vi "PPMS_Data_Recorder2.vi"(1 "Output Amp #1":dbl=1.0, 2 "Output Amp #2":dbl=1.0, 3 "Output Amp #3":dbl=1.0) -> (7 "X-Value":dbl, 8 "X-Value 2":dbl, 9 "Theta-Value":dbl, 10 "Theta-Value 2":dbl)   [LabVIEW 2021]
uses:
  <instrlib>/Stanford Research 830/Public/Data/Read (All Parameters).vi
  \\ad.monash.edu\home/User060/c-nhppms/Desktop/Matt Gebert/LabViewPrograms/3rd Party Drivers/QDI-PPMS/QDInstrument.dll
  3rd Party Drivers/QDI-PPMS/QDInstrument.dll
  <instrlib>/Stanford Research 830/Stanford Research 830.lvlib
panel:
  in  "Data Format String":string="%.12f"
  out "Actual Save Path":path
  in  "File Notes:":string
  in  "<File Name>.dat  (Don't add extension)":string
  in  "Data Save Path:":path=path "C:/Users/labpc/Documents/ProbeStation Users Data"
  in  "Record data to file?":bool
  out "Temperature":dbl
  out "Field":dbl
  out "PPMS Initialisation":bool
  in  "Remote":bool
  out "PPMS Chamber Status":i32(ring) items=["ChamberUnknown"=0, "PurgedAndSealed"=1, "VentedAndSealed"=2, "Sealed"=3, "Purging"=4, "Venting"=5, "PreHiVac"=6, "HighVac"=7, "PumpContinuous"=8, "VentContinuous"=9, "ChamberFailure"=15]
  in  "External Reference Trigger (0: Sine Zero Crossing)  2":u16(ring) items=["Sine Zero Crossing", "TTL Rising Edge", "TTL Falling Edge"]
  in  "External Reference Trigger (0: Sine Zero Crossing)":u16(ring) items=["Sine Zero Crossing", "TTL Rising Edge", "TTL Falling Edge"]
  in  "External Reference Trigger #2 (0: Sine Zero Crossing)":u16(ring) items=["Sine Zero Crossing", "TTL Rising Edge", "TTL Falling Edge"]
  out "SR830 #3 Sensitivity 3":dbl
  out "SR830 #3 Sensitivity 2":dbl
  out "SR830 #3 Sensitivity":dbl
  out "Sense\nOver 3":bool
  out "Sense\nUnder 3":bool
  out "Sense\nOver 2":bool
  out "Sense\nUnder 2":bool
  out "Sense Under":bool
  out "Sense Over":bool
  in  "Loop Timing (ms)":u32=500
  out "Reference Freq 3":dbl
  out "Theta-Value 3":dbl
  out "R-Value 3":dbl
  out "X-Value 3":dbl
  out "Reference Freq 2":dbl
  out "R-Value 2":dbl
  out "Reference Freq":dbl
  out "R-Value":dbl
  out "Device Intialization":T1
  in  "System #3 Enabled/Disabled":bool
  in  "SR830 #3":refnum<visa-resource-name>="GPIB0::10::INSTR"
  in  "SR830 #3 Input Connection":u16(ring) items=["Single-Ended Voltage", "Differential Voltage", "1 MOhm Current Gain", "100 MOhm Current Gain"]
  in  "SR830 #3\nInput Coupling":u16(ring) items=["AC", "DC"]
  in  "SR830 #3 Input \nShield Grounding":u16(ring) items=["Float", "Ground"]
  in  "SR830 #3 Input\nNotch Filter":u16(ring) items=["None", "Line Notch", "2x Line Notch", "Both Notch Filters"]
  in  "SR830 #3 Trigger Source":u16(ring) items=["Internal", "External"]
  in  "SR830 #3 Internal \nReference Frequency":dbl=17.0
  in  "SR830 #3 Detection Harm. Num.":dbl=1.0
  in  "SR830 #3 Reference Source":u16(ring) items=["External", "Internal"]
  in  "SR830 #3 Manual \nPhase":dbl
  in  "SR830 #3 \nAuto Phase":bool
  in  "SR830 #3 \nTime Constant":u16(ring)=9 items=["10 us", "30 us", "100 us", "300 us", "1 ms", "3 ms", "10 ms", "30 ms", "100 ms", "300 ms", "1 s", "3 s", "10 s", "30 s", "100 s", "300 s", "1 ks", "3 ks", "10 ks", "30 ks"]
  in  "SR830 #3 Low\nPass Filter Slope":u16(ring)=3 items=["6 dB/oct", "12 dB/oct", "18 db/oct", "24 dB/oct"]
  in  "SR830 #3\nSync Filter":bool
  in  "SR830 #3 \nDynamic Reserve":i16(ring)=1 items=["Auto Reserve"=-1, "High Reserve"=0, "Normal"=1, "Low Noise"=2]
  in  "SR830 #3 Initial\nSensitivity":i16(ring)=17 items=["Auto Gain"=-1, "2 nV/fA"=0, "5 nV/fA"=1, "10 nV/fA"=2, "20 nV/fA"=3, "50 nV/fA"=4, "100 nV/fA"=5, "200 nV/fA"=6, "500 nV/fA"=7, "1 uV/pA"=8, "2 uV/pA"=9, "5 uV/pA"=10, "10 uV/pA"=11, "20 uV/pA"=12, "50 uV/pA"=13, "100 uV/pA"=14, "200 uV/pA"=15, "500 uV/pA"=16, "1 mV/nA"=17, "2 mV/nA"=18, "5 mV/nA"=19, "10 mV/nA"=20, "20 mV/nA"=21, "50 mV/nA"=22, "100 mV/nA"=23, "200 mV/nA"=24, "500 mV/mA"=25, "1 V/uA"=26]
  in  "System #2 Enabled/Disabled":bool
  in  "SR830 #2":refnum<visa-resource-name>="GPIB0::10::INSTR"
  in  "SR830 #2 Input Connection":u16(ring)=1 items=["Single-Ended Voltage", "Differential Voltage", "1 MOhm Current Gain", "100 MOhm Current Gain"]
  in  "SR830 #2\nInput Coupling":u16(ring) items=["AC", "DC"]
  in  "SR830 #2 Input \nShield Grounding":u16(ring) items=["Float", "Ground"]
  in  "SR830 #2 Input\nNotch Filter":u16(ring) items=["None", "Line Notch", "2x Line Notch", "Both Notch Filters"]
  in  "SR830 #2 Trigger Source":u16(ring) items=["Internal", "External"]
  in  "SR830 #2 Internal \nReference Frequency":dbl=17.0
  in  "SR830 #2 Detection Harm. Num.":dbl=1.0
  in  "SR830 #2 Reference Source":u16(ring) items=["External", "Internal"]
  in  "SR830 #2 Manual \nPhase":dbl
  in  "SR830 #2 \nAuto Phase":bool
  in  "SR830 #2 \nTime Constant":u16(ring)=8 items=["10 us", "30 us", "100 us", "300 us", "1 ms", "3 ms", "10 ms", "30 ms", "100 ms", "300 ms", "1 s", "3 s", "10 s", "30 s", "100 s", "300 s", "1 ks", "3 ks", "10 ks", "30 ks"]
  in  "SR830 #2 Low\nPass Filter Slope":u16(ring)=3 items=["6 dB/oct", "12 dB/oct", "18 db/oct", "24 dB/oct"]
  in  "SR830 #2\nSync Filter":bool
  in  "SR830 #2 \nDynamic Reserve":i16(ring)=1 items=["Auto Reserve"=-1, "High Reserve"=0, "Normal"=1, "Low Noise"=2]
  in  "SR830 #2 Initial \nSensitivity":i16(ring)=17 items=["Auto Gain"=-1, "2 nV/fA"=0, "5 nV/fA"=1, "10 nV/fA"=2, "20 nV/fA"=3, "50 nV/fA"=4, "100 nV/fA"=5, "200 nV/fA"=6, "500 nV/fA"=7, "1 uV/pA"=8, "2 uV/pA"=9, "5 uV/pA"=10, "10 uV/pA"=11, "20 uV/pA"=12, "50 uV/pA"=13, "100 uV/pA"=14, "200 uV/pA"=15, "500 uV/pA"=16, "1 mV/nA"=17, "2 mV/nA"=18, "5 mV/nA"=19, "10 mV/nA"=20, "20 mV/nA"=21, "50 mV/nA"=22, "100 mV/nA"=23, "200 mV/nA"=24, "500 mV/mA"=25, "1 V/uA"=26]
  in  "SR830 #1 Initial\nSensitivity":i16(ring)=17 items=["Auto Gain"=-1, "2 nV/fA"=0, "5 nV/fA"=1, "10 nV/fA"=2, "20 nV/fA"=3, "50 nV/fA"=4, "100 nV/fA"=5, "200 nV/fA"=6, "500 nV/fA"=7, "1 uV/pA"=8, "2 uV/pA"=9, "5 uV/pA"=10, "10 uV/pA"=11, "20 uV/pA"=12, "50 uV/pA"=13, "100 uV/pA"=14, "200 uV/pA"=15, "500 uV/pA"=16, "1 mV/nA"=17, "2 mV/nA"=18, "5 mV/nA"=19, "10 mV/nA"=20, "20 mV/nA"=21, "50 mV/nA"=22, "100 mV/nA"=23, "200 mV/nA"=24, "500 mV/mA"=25, "1 V/uA"=26]
  in  "SR830 #1 \nDynamic Reserve":i16(ring)=1 items=["Auto Reserve"=-1, "High Reserve"=0, "Normal"=1, "Low Noise"=2]
  in  "SR830 #1\nSync Filter":bool
  in  "SR830 #1 Low\nPass Filter Slope":u16(ring)=3 items=["6 dB/oct", "12 dB/oct", "18 db/oct", "24 dB/oct"]
  in  "SR830 #1 \nTime Constant":u16(ring)=8 items=["10 us", "30 us", "100 us", "300 us", "1 ms", "3 ms", "10 ms", "30 ms", "100 ms", "300 ms", "1 s", "3 s", "10 s", "30 s", "100 s", "300 s", "1 ks", "3 ks", "10 ks", "30 ks"]
  in  "SR830 #1 \nAuto Phase":bool
  in  "SR830 #1 Manual \nPhase":dbl
  in  "SR830 #1 Reference Source":u16(ring)=1 items=["External", "Internal"]
  in  "SR830 #1 Detection Harm. Num.":dbl=1.0
  in  "SR830 #1 Internal \nReference Frequency":dbl=17.0
  in  "SR830 #1 Trigger Source":u16(ring) items=["Internal", "External"]
  in  "SR830 #1 Input\nNotch Filter":u16(ring) items=["None", "Line Notch", "2x Line Notch", "Both Notch Filters"]
  in  "SR830 #1 Input \nShield Grounding":u16(ring) items=["Float", "Ground"]
  in  "SR830 #1\nInput Coupling":u16(ring) items=["AC", "DC"]
  in  "SR830 #1 Input Connection":u16(ring)=1 items=["Single-Ended Voltage", "Differential Voltage", "1 MOhm Current Gain", "100 MOhm Current Gain"]
  in  "SR830 #1":refnum<visa-resource-name>="GPIB0::10::INSTR"
  in  "System #1 Enabled/Disabled":bool
  in  "System Reset All?":bool
  in  "program_stop":bool
  out "Y-Value 3":dbl
  out "Y-Value 2":dbl
  out "Y-Value":dbl
  # "Readout (Recorded)"
  # "SR830"
  # "SR830"
  # "SR830"
  # "Input Signal"
  # "Input Signal"
  # "Input Signal"
  # "Readout (Recorded)"
  # "Readout (Recorded)"
  # "Source / Reference"
  # "Source / Reference"
  # "Source / Reference"
  # "Input Filters & Sens"
  # "Input Filters & Sens"
  # "Input Filters & Sens"
  # "Initialisation:\n--> Reset \n--> Instruments?"
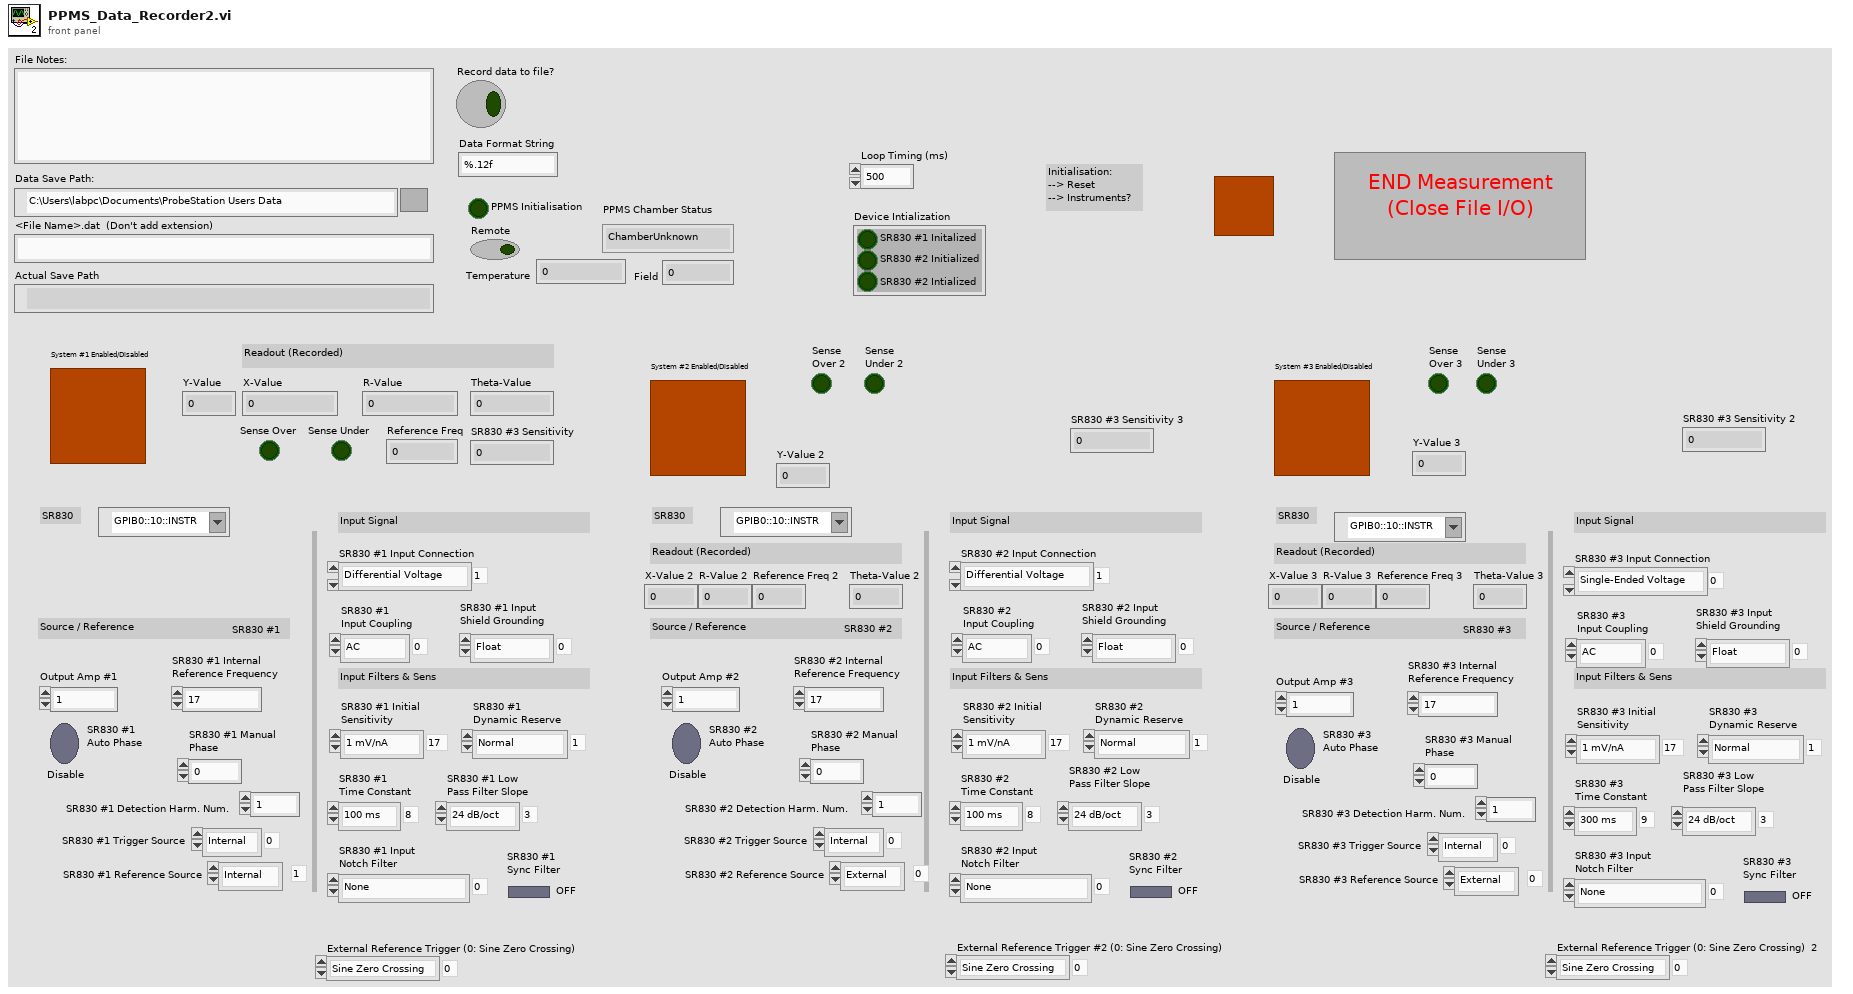
[diagram p1: front panel]
types:
  T1 = cluster{"SR830 #1 Initalized":bool, "SR830 #2 Initialized":bool, "SR830 #2 Intialized":bool}
  T2 = cluster{"Instrument Ref Out":refnum<k24>, "error out":errorcluster}
  T3 = cluster{"VISA resource name out":refnum<visa-resource-name>, "error out":errorcluster}
  T4 = cluster{"Initialised?":bool, "Initialised?":bool, "Initialised?":bool}
  T5 = cluster{"RecordingInProgress":bool, "refnum out":refnum<file>, "error out":errorcluster, "Actual Save Path":path}
  T6 = cluster{"Reference & Errors":cluster{"VISA resource name out":refnum<visa-resource-name>, "error out":errorcluster}, "Reference & Errors":cluster{"VISA resource name out":refnum<visa-resource-name>, "error out":errorcluster}, "Reference & Errors":cluster{"VISA resource name out":refnum<visa-resource-name>, "error out":errorcluster}}
  T7 = cluster{"Voltage Output":dbl, "Voltage Output":dbl, "Voltage Output":dbl}
  T8 = cluster{"Sensitivity":i16, "Sensitivity":i16, "Sensitivity":i16}
  T9 = cluster{"System #1 Enabled/Disabled":bool, "System #2 Enabled/Disabled":bool, "System #3 Enabled/Disabled":bool}
  T10 = cluster{"X-Value":dbl, "Y-Value":dbl, "R-Value":dbl, "Theta-Value":dbl, "Aux In 1 Value":dbl, "Aux In 2 Value":dbl, "Aux In 3 Value":dbl, "Aux In 4 Value":dbl, "Reference Frequency":dbl, "Channel 1 Display":dbl, "Channel 2 Display":dbl}
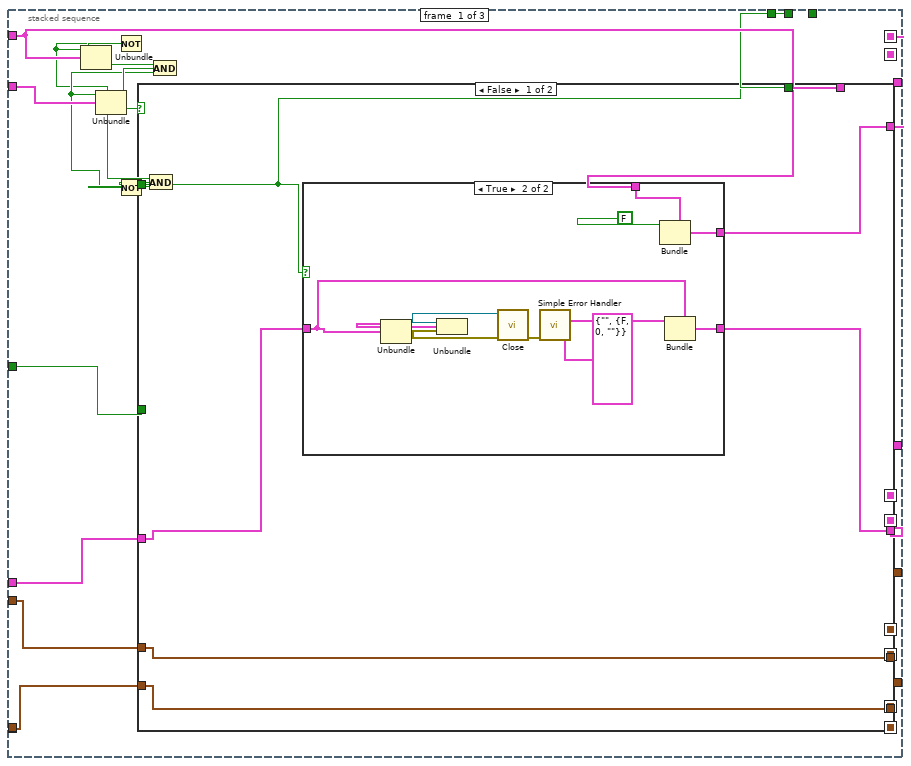
[diagram p6: hidden frame]
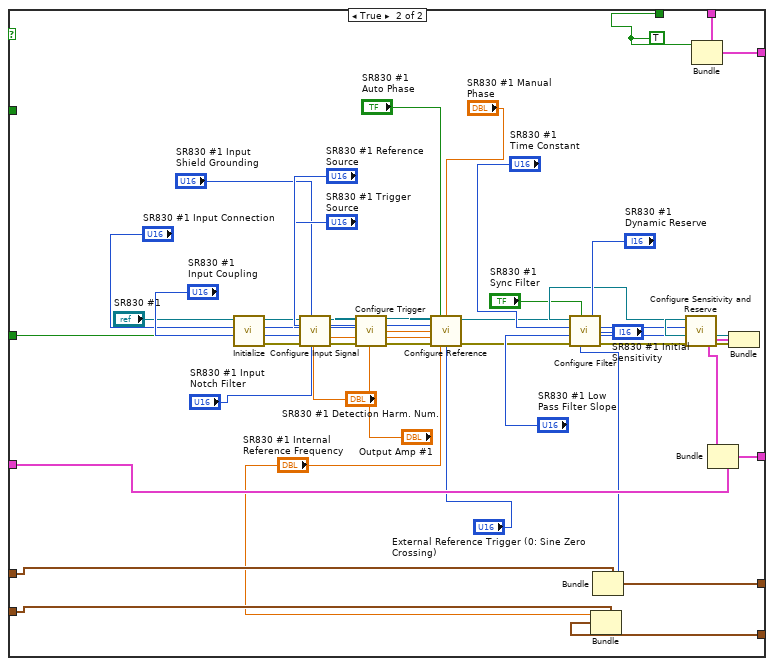
[diagram p8: hidden frame]
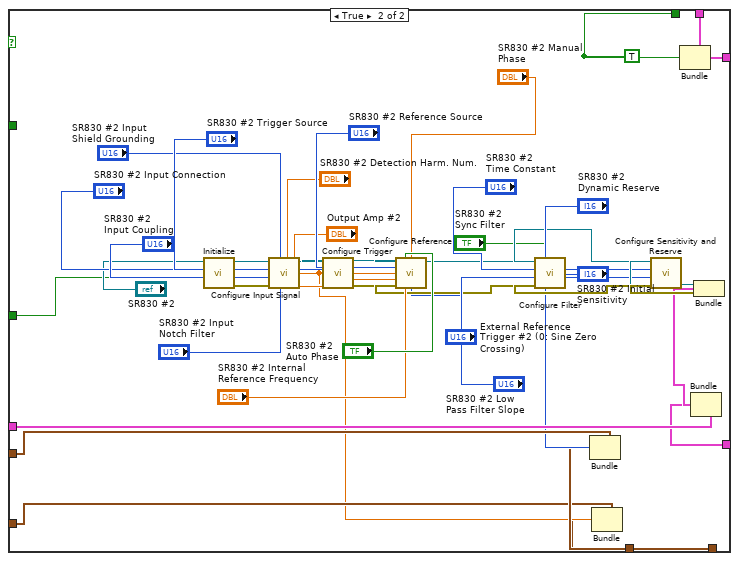
[diagram p10: hidden frame]
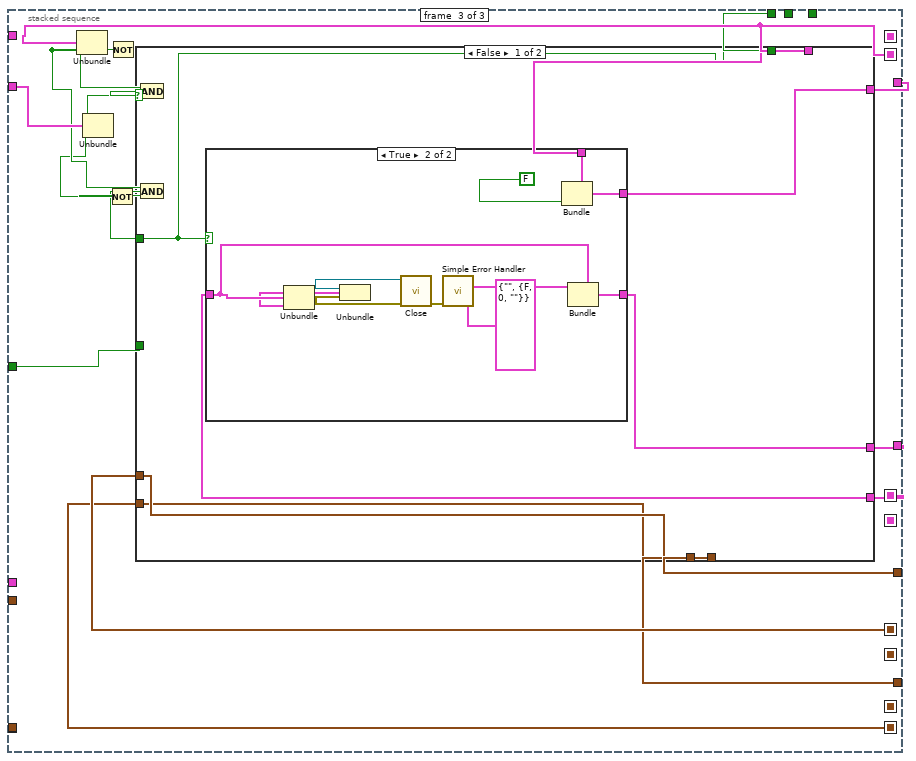
[diagram p11: hidden frame]
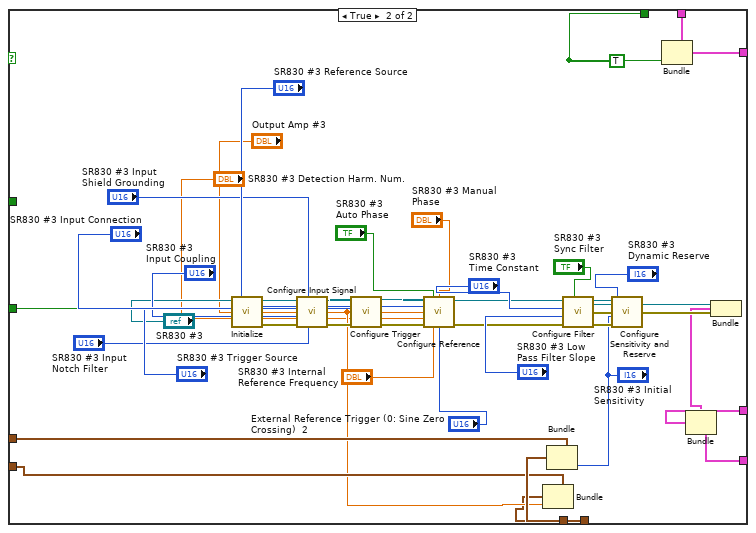
[diagram p13: hidden frame]
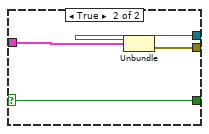
[diagram p14: hidden frame]
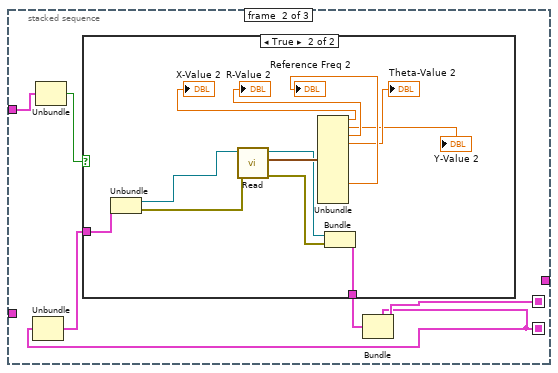
[diagram p16: hidden frame]
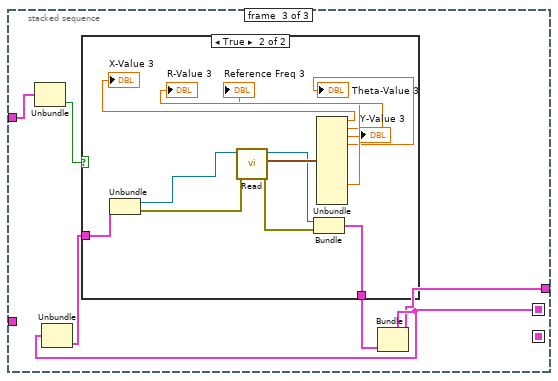
[diagram p18: hidden frame]
diagram:
  w5 = path ""  # Actual Save Path
  w9 = FALSE  # RecordingInProgress
  (unwired) FALSE  # File Init
  w10 = T2 {"Instrument Ref Out"=refnum, "error out"={"status"=FALSE, "code"=0, "source"=""}}  # PPMS Status Cluster
  w11 = FALSE  # PPMS Init
  w14 = 0.0 ("Voltage Output")
  w15 = i16 17 items=["Auto Gain"=-1, "2 nV/fA"=0, "5 nV/fA"=1, "10 nV/fA"=2, "20 nV/fA"=3, "50 nV/fA"=4, "100 nV/fA"=5, "200 nV/fA"=6, "500 nV/fA"=7, "1 uV/pA"=8, "2 uV/pA"=9, "5 uV/pA"=10, "10 uV/pA"=11, "20 uV/pA"=12, "50 uV/pA"=13, "100 uV/pA"=14, "200 uV/pA"=15, "500 uV/pA"=16, "1 mV/nA"=17, "2 mV/nA"=18, "5 mV/nA"=19, "10 mV/nA"=20, "20 mV/nA"=21, "50 mV/nA"=22, "100 mV/nA"=23, "200 mV/nA"=24, "500 mV/mA"=25, "1 V/uA"=26] ("Sensitivity")
  w25 = T3 {"VISA resource name out"="", "error out"={"status"=FALSE, "code"=0, "source"=""}} ("Reference & Errors")
  w27 = FALSE ("Initialised?")
  (unwired) ".txt"
  (unwired) FALSE ("Measuring")
  n1 = Bundle("Initialised?"=w27, "Initialised?"=w27, "Initialised?"=w27) -> (w26:T4)  [unwired: 1 in]
  n2 = Bundle("RecordingInProgress"=w9, "refnum out"=refnum<file> refnum, "error out"=errorcluster {"status"=FALSE, "code"=0, "source"=""}, "Actual Save Path"=w5) -> (w8:T5)  [unwired: 1 in]
  n3 = Bundle("Reference & Errors"=w25, "Reference & Errors"=w25, "Reference & Errors"=w25) -> (w24:T6)  [unwired: 1 in]
  n4 = Bundle("Voltage Output"=w14, "Voltage Output"=w14, "Voltage Output"=w14) -> (w13:T7)  [unwired: 1 in]
  n5 = Bundle("Sensitivity"=w15, "Sensitivity"=w15, "Sensitivity"=w15) -> (w12:T8)  [unwired: 1 in]
  n6 = while {
    shift-right: [w59] -> w23
    shift-left: w26 -> [w62]
    shift-right: [w48] -> w22
    shift-left: w24 -> [w47]
    shift-right: [w56] -> _
    shift-left: w12 -> [w58]
    shift-right: [w49] -> _
    shift-left: w13 -> [w53]
    shift-right: [w45] -> _
    shift-left: w11 -> [w46]
    shift-right: [w41] -> _
    shift-left: w10 -> [w43]
    shift-right: [w29] -> w4
    shift-left: w8 -> [w30]
    stop <- "program_stop" stop-if-true
    n7 = flat-sequence {
      tunnel: w62 -> [w80]
      tunnel: w47 -> [w79]
      tunnel: [w77] -> w61
      tunnel: [w78] -> w60
      tunnel: [w78] -> w59
      tunnel: w58 -> [w76]
      tunnel: [w75] -> w57
      tunnel: w53 -> [w74]
      tunnel: [w73] -> w52
      tunnel: w46 -> [w68]
      tunnel: [w67] -> w45
      tunnel: w43 -> [w66]
      tunnel: [w65] -> w42
      tunnel: [w64] -> w32
      tunnel: w61 -> [w374]
      tunnel: w60 -> [w373]
      tunnel: [w375] -> w40
      tunnel: w57 -> [w377]
      tunnel: [w377] -> w38
      tunnel: [w373] -> w36
      tunnel: w52 -> [w376]
      tunnel: [w376] -> w34
      tunnel: w42 -> [w372]
      tunnel: [w371] -> w41
      tunnel: w32 -> [w370]
      tunnel: [w370] -> w31
      tunnel: w40 -> [w457]
      tunnel: [w457] -> w39
      tunnel: w38 -> [w456]
      tunnel: [w456] -> w37
      tunnel: w36 -> [w450]
      tunnel: [w450] -> w35
      tunnel: w34 -> [w455]
      tunnel: [w455] -> w33
      tunnel: w31 -> [w454]
      tunnel: w30 -> [w449]
      tunnel: [w448] -> w29
      tunnel: w39 -> [w637]
      tunnel: w37 -> [w640]
      tunnel: [w640] -> w55
      tunnel: w35 -> [w638]
      tunnel: [w638] -> w54
      tunnel: w33 -> [w639]
      tunnel: [w636] -> w51
      tunnel: [w635] -> w50
      tunnel: w55 -> [w739]
      tunnel: [w738] -> w56
      tunnel: [w737] -> w48
      tunnel: w54 -> [w736]
      tunnel: w51 -> [w729]
      tunnel: w50 -> [w728]
      tunnel: [w728] -> w49
      frame #0 {
        # "Device Initialization or close"
        n8 = flat-sequence {
          tunnel: w80 -> [w97]
          tunnel: w79 -> [w96]
          tunnel: w76 -> [w93]
          tunnel: w74 -> [w91]
          tunnel: [w95] -> w72
          tunnel: [w94] -> w71
          tunnel: [w92] -> w70
          tunnel: [w90] -> w69
          tunnel: [w81] -> w64
          tunnel: [w339] -> w73
          tunnel: [w340] -> w75
          tunnel: [w341] -> w77
          tunnel: [w342] -> w78
          tunnel: w72 -> [w342]
          tunnel: w71 -> [w341]
          tunnel: w70 -> [w340]
          tunnel: w69 -> [w339]
          tunnel: w68 -> [w338]
          tunnel: [w337] -> w67
          tunnel: w66 -> [w331]
          tunnel: [w330] -> w65
          frame #0 {
            # "SR830 Lock In Amplifiers"
            n9 = Bundle("System #1 Enabled/Disabled"="System #1 Enabled/Disabled", "System #2 Enabled/Disabled"="System #2 Enabled/Disabled", "System #3 Enabled/Disabled"="System #3 Enabled/Disabled") -> (w87:T9)  [unwired: 1 in]
            n10 = stacked-sequence {
              seq-local: [w110 _ _] -> [_ w188 _]
              seq-local: [_ w187 _] -> [_ _ w265]
              seq-local: [w109 _ _] -> [_ w186 _]
              seq-local: [_ w185 _] -> [_ _ w263]
              seq-local: [w102 _ _] -> [_ w180 _]
              seq-local: [_ w179 _] -> [_ _ w257]
              seq-local: [_ w177 _] -> [_ _ w255]
              seq-local: [w100 _ _] -> [_ w178 _]
              tunnel: "System Reset All?" -> [w115 w192 w269]
              tunnel: w87 -> [w114 w191 w267]
              tunnel: w97 -> [w111 _ _]
              tunnel: w96 -> [w104 _ _]
              tunnel: [_ _ w264] -> w95
              tunnel: [_ _ w262] -> w94
              tunnel: w93 -> [w103 _ _]
              tunnel: [_ _ w256] -> w92
              tunnel: [w101 _ _] -> _
              tunnel: w91 -> [w101 _ _]
              tunnel: [_ _ w254] -> w90
              tunnel: [_ _ w253] -> w84
              tunnel: [w99 _ _] -> w83
              tunnel: [_ w176 _] -> w82
              frame #0 {
                n11 = Unbundle(w111) -> ("Initialised?"=w106:bool)  [unwired: 2 out]
                n12 = Unbundle(w114) -> ("System #1 Enabled/Disabled"=w107:bool)  [unwired: 2 out]
                n13 = Not(x=w106) -> (.not. x?=w113:bool)
                n14 = Not(x=w107) -> (.not. x?=w108:bool)
                n15 = And(x=w106, y=w108) -> (x .and. y?=w105:bool)
                n16 = And(x=w113, y=w107) -> (x .and. y?=w112:bool)
                n17 = case shown="False" w112 {
                  tunnel: w115 -> [_ w148]
                  tunnel: w111 -> [w120 w147]
                  tunnel: [w119 w146] -> w110
                  tunnel: w104 -> [w122 w145]
                  tunnel: [w121 w143] -> w109
                  tunnel: w105 -> [w116 _]
                  tunnel: w103 -> [w118 w142]
                  tunnel: [w118 w141] -> w102
                  tunnel: w101 -> [w117 w139]
                  tunnel: [w117 w138] -> w100
                  tunnel: [w116 w135] -> w99
                  frame False {
                    n18 = case shown="True" w116 {
                      tunnel: w122 -> [w124 w131]
                      tunnel: [w124 w129] -> w121
                      tunnel: w120 -> [w123 w126]
                      tunnel: [w123 w125] -> w119
                      frame False {
                      }
                      frame True {
                        n19 = Unbundle(w131) -> ("Reference & Errors"=w128:T3)  [unwired: 2 out]
                        n20 = Unbundle(w128) -> ("VISA resource name out"=w133:refnum<visa-resource-name>, "error out"=w132:errorcluster)
                        n21 = call <instrlib>:"Close.vi"("error in (no error)"=w132, "VISA resource name"=w133) -> ("error out"=w134:errorcluster)  [unwired: 9 in]
                        n22 = call <vilib>:"Simple Error Handler.vi"("error in (no error)"=w134) -> ()  [unwired: 4 in, 5 out]
                        n23 = Bundle(cluster=w126, "Initialised?"=FALSE) -> (w125:T4)  [unwired: 2 in]
                        n24 = Bundle(cluster=w131, "Reference & Errors"=T3 {"VISA resource name out"="", "error out"={"status"=FALSE, "code"=0, "source"=""}}) -> (w129:T6)  [unwired: 2 in]
                      }
                    }
                  }
                  frame True {
                    w135 = TRUE
                    n25 = call <instrlib>:"Initialize.vi"("Reset (True)"=w148, "VISA resource name"="SR830 #1") -> ("error out"=w153:errorcluster, "VISA resource name out"=w152:refnum<visa-resource-name>)  [unwired: 8 in]
                    n26 = call <instrlib>:"Configure Input Signal.vi"("Input Notch Filter (0: None)"="SR830 #1 Input\nNotch Filter", "Input Shield Grounding (0: Float)"="SR830 #1 Input \nShield Grounding", "error in (no error)"=w153, "Input Coupling (0: AC)"="SR830 #1\nInput Coupling", "Input Connection (0: Single-Ended Voltage)"="SR830 #1 Input Connection", "VISA resource name"=w152) -> ("error out"=w155:errorcluster, "VISA resource name out"=w154:refnum<visa-resource-name>)  [unwired: 4 in]
                    n27 = call <instrlib>:"Configure Trigger.vi"("error in (no error)"=w155, "Trigger Source (0: Internal)"="SR830 #1 Trigger Source", "VISA resource name"=w154) -> ("error out"=w157:errorcluster, "VISA resource name out"=w156:refnum<visa-resource-name>)  [unwired: 7 in]
                    n28 = call <instrlib>:"Configure Reference.vi"("VISA resource name"=w156, "Auto Phase (T: Enabled)"="SR830 #1 \nAuto Phase", "Manual Phase (0 Degree)"="SR830 #1 Manual \nPhase", "Reference Source (1: Internal)"="SR830 #1 Reference Source", "Sine Output Amplitude (1 V)"="Output Amp #1", "Detection Harmonic Number (1)"="SR830 #1 Detection Harm. Num.", "error in (no error)"=w157, "Internal Reference Frequency (1000 Hz)"="SR830 #1 Internal \nReference Frequency", "External Reference Trigger (0: Sine Zero Crossing)"="External Reference Trigger (0: Sine Zero Crossing)") -> ("VISA resource name out"=w159:refnum<visa-resource-name>, "error out"=w158:errorcluster)  [unwired: 5 in]
                    n29 = call <instrlib>:"Configure Filter.vi"("Enable Sync Filter (F: Disable)"="SR830 #1\nSync Filter", "error in (no error)"=w158, "Low Pass Filter Slope (1: 12dB/oct)"="SR830 #1 Low\nPass Filter Slope", "Time Constant (8: 100ms)"="SR830 #1 \nTime Constant", "VISA resource name"=w159) -> ("error out"=w172:errorcluster, "VISA resource name out"=w171:refnum<visa-resource-name>)  [unwired: 5 in]
                    n30 = Bundle(cluster=w139, "Voltage Output"="SR830 #1 Internal \nReference Frequency") -> (w138:T7)  [unwired: 2 in]
                    n31 = Bundle(cluster=w142, "Sensitivity"="SR830 #1 Initial\nSensitivity") -> (w141:T8)  [unwired: 2 in]
                    n32 = call <instrlib>:"Configure Sensitivity and Reserve.vi"("error in (no error)"=w172, "Sensitivity (-1: Auto gain)"="SR830 #1 Initial\nSensitivity", "Dynamic Reserve (-1: Auto Reserve)"="SR830 #1 \nDynamic Reserve", "VISA resource name"=w171) -> ("error out"=w175:errorcluster, "VISA resource name out"=w174:refnum<visa-resource-name>)  [unwired: 6 in]
                    n33 = Bundle(cluster=w147, "Initialised?"=w135) -> (w146:T4)  [unwired: 2 in]
                    n34 = Bundle("VISA resource name out"=w174, "error out"=w175) -> (w144:T3)  [unwired: 1 in]
                    n35 = Bundle(cluster=w145, "Reference & Errors"=w144) -> (w143:T6)  [unwired: 2 in]
                  }
                }
              }
              frame #1 {
                n36 = Unbundle(w188) -> ("Initialised?"=w182:bool)  [unwired: 2 out]
                n37 = Unbundle(w191) -> ("System #2 Enabled/Disabled"=w181:bool)  [unwired: 2 out]
                n38 = Not(x=w181) -> (.not. x?=w184:bool)
                n39 = And(x=w182, y=w184) -> (x .and. y?=w183:bool)
                n40 = Not(x=w182) -> (.not. x?=w190:bool)
                n41 = And(x=w190, y=w181) -> (x .and. y?=w189:bool)
                n42 = case shown="False" w189 {
                  tunnel: w192 -> [_ w225]
                  tunnel: w188 -> [w197 w224]
                  tunnel: [w196 w223] -> w187
                  tunnel: w186 -> [w199 w221]
                  tunnel: [w198 w220] -> w185
                  tunnel: w183 -> [w193 _]
                  tunnel: w180 -> [w195 w219]
                  tunnel: [w195 w217] -> w179
                  tunnel: w178 -> [w194 w216]
                  tunnel: [w194 w214] -> w177
                  tunnel: [w193 w212] -> w176
                  frame False {
                    n43 = case shown="True" w193 {
                      tunnel: w199 -> [w201 w208]
                      tunnel: [w201 w206] -> w198
                      tunnel: w197 -> [w200 w204]
                      tunnel: [w200 w203] -> w196
                      frame False {
                      }
                      frame True {
                        n44 = Unbundle(w208) -> ("Reference & Errors"=w205:T3)  [unwired: 2 out]
                        n45 = Unbundle(w205) -> ("VISA resource name out"=w210:refnum<visa-resource-name>, "error out"=w209:errorcluster)
                        n46 = call <instrlib>:"Close.vi"("error in (no error)"=w209, "VISA resource name"=w210) -> ("error out"=w211:errorcluster)  [unwired: 9 in]
                        n47 = call <vilib>:"Simple Error Handler.vi"("error in (no error)"=w211) -> ()  [unwired: 4 in, 5 out]
                        n48 = Bundle(cluster=w208, "Reference & Errors"=T3 {"VISA resource name out"="", "error out"={"status"=FALSE, "code"=0, "source"=""}}) -> (w206:T6)  [unwired: 2 in]
                        n49 = Bundle(cluster=w204, "Initialised?"=FALSE) -> (w203:T4)  [unwired: 2 in]
                      }
                    }
                  }
                  frame True {
                    w212 = TRUE
                    n50 = call <instrlib>:"Initialize.vi"("Reset (True)"=w225, "VISA resource name"="SR830 #2") -> ("error out"=w230:errorcluster, "VISA resource name out"=w229:refnum<visa-resource-name>)  [unwired: 8 in]
                    n51 = call <instrlib>:"Configure Input Signal.vi"("Input Notch Filter (0: None)"="SR830 #2 Input\nNotch Filter", "Input Shield Grounding (0: Float)"="SR830 #2 Input \nShield Grounding", "error in (no error)"=w230, "Input Coupling (0: AC)"="SR830 #2\nInput Coupling", "Input Connection (0: Single-Ended Voltage)"="SR830 #2 Input Connection", "VISA resource name"=w229) -> ("error out"=w232:errorcluster, "VISA resource name out"=w231:refnum<visa-resource-name>)  [unwired: 4 in]
                    n52 = call <instrlib>:"Configure Trigger.vi"("error in (no error)"=w232, "Trigger Source (0: Internal)"="SR830 #2 Trigger Source", "VISA resource name"=w231) -> ("error out"=w234:errorcluster, "VISA resource name out"=w233:refnum<visa-resource-name>)  [unwired: 7 in]
                    n53 = call <instrlib>:"Configure Reference.vi"("VISA resource name"=w233, "Auto Phase (T: Enabled)"="SR830 #2 \nAuto Phase", "Manual Phase (0 Degree)"="SR830 #2 Manual \nPhase", "Reference Source (1: Internal)"="SR830 #2 Reference Source", "Sine Output Amplitude (1 V)"="Output Amp #2", "Detection Harmonic Number (1)"="SR830 #2 Detection Harm. Num.", "error in (no error)"=w234, "Internal Reference Frequency (1000 Hz)"="SR830 #2 Internal \nReference Frequency", "External Reference Trigger (0: Sine Zero Crossing)"="External Reference Trigger #2 (0: Sine Zero Crossing)") -> ("VISA resource name out"=w236:refnum<visa-resource-name>, "error out"=w235:errorcluster)  [unwired: 5 in]
                    n54 = call <instrlib>:"Configure Filter.vi"("Enable Sync Filter (F: Disable)"="SR830 #2\nSync Filter", "error in (no error)"=w235, "Low Pass Filter Slope (1: 12dB/oct)"="SR830 #2 Low\nPass Filter Slope", "Time Constant (8: 100ms)"="SR830 #2 \nTime Constant", "VISA resource name"=w236) -> ("error out"=w249:errorcluster, "VISA resource name out"=w248:refnum<visa-resource-name>)  [unwired: 5 in]
                    n55 = Bundle(cluster=w219, "Sensitivity"="SR830 #2 Initial \nSensitivity") -> (w217:T8)  [unwired: 2 in]
                    n56 = Bundle(cluster=w216, "Voltage Output"="Output Amp #2") -> (w214:T7)  [unwired: 2 in]
                    n57 = call <instrlib>:"Configure Sensitivity and Reserve.vi"("error in (no error)"=w249, "Sensitivity (-1: Auto gain)"="SR830 #2 Initial \nSensitivity", "Dynamic Reserve (-1: Auto Reserve)"="SR830 #2 \nDynamic Reserve", "VISA resource name"=w248) -> ("error out"=w252:errorcluster, "VISA resource name out"=w251:refnum<visa-resource-name>)  [unwired: 6 in]
                    n58 = Bundle(cluster=w224, "Initialised?"=w212) -> (w223:T4)  [unwired: 2 in]
                    n59 = Bundle("VISA resource name out"=w251, "error out"=w252) -> (w222:T3)  [unwired: 1 in]
                    n60 = Bundle(cluster=w221, "Reference & Errors"=w222) -> (w220:T6)  [unwired: 2 in]
                  }
                }
              }
              frame #2 {
                n61 = Unbundle(w265) -> ("Initialised?"=w260:bool)  [unwired: 2 out]
                n62 = Unbundle(w267) -> ("System #3 Enabled/Disabled"=w259:bool)  [unwired: 2 out]
                n63 = Not(x=w259) -> (.not. x?=w261:bool)
                n64 = Not(x=w260) -> (.not. x?=w268:bool)
                n65 = And(x=w268, y=w259) -> (x .and. y?=w266:bool)
                n66 = And(x=w260, y=w261) -> (x .and. y?=w258:bool)
                n67 = case shown="False" w266 {
                  tunnel: w269 -> [_ w303]
                  tunnel: w265 -> [w274 w302]
                  tunnel: [w273 w301] -> w264
                  tunnel: w258 -> [w270 _]
                  tunnel: w263 -> [w276 w300]
                  tunnel: [w275 w299] -> w262
                  tunnel: w257 -> [w272 w297]
                  tunnel: [w272 w296] -> w256
                  tunnel: w255 -> [w271 w294]
                  tunnel: [w271 w292] -> w254
                  tunnel: [w270 w289] -> w253
                  frame False {
                    n68 = case shown="True" w270 {
                      tunnel: w276 -> [w278 w285]
                      tunnel: [w278 w283] -> w275
                      tunnel: w274 -> [w277 w281]
                      tunnel: [w277 w280] -> w273
                      frame False {
                      }
                      frame True {
                        n69 = Unbundle(w285) -> ("Reference & Errors"=w282:T3)  [unwired: 2 out]
                        n70 = Unbundle(w282) -> ("VISA resource name out"=w287:refnum<visa-resource-name>, "error out"=w286:errorcluster)
                        n71 = call <instrlib>:"Close.vi"("error in (no error)"=w286, "VISA resource name"=w287) -> ("error out"=w288:errorcluster)  [unwired: 9 in]
                        n72 = call <vilib>:"Simple Error Handler.vi"("error in (no error)"=w288) -> ()  [unwired: 4 in, 5 out]
                        n73 = Bundle(cluster=w281, "Initialised?"=FALSE) -> (w280:T4)  [unwired: 2 in]
                        n74 = Bundle(cluster=w285, "Reference & Errors"=T3 {"VISA resource name out"="", "error out"={"status"=FALSE, "code"=0, "source"=""}}) -> (w283:T6)  [unwired: 2 in]
                      }
                    }
                  }
                  frame True {
                    w289 = TRUE
                    n75 = call <instrlib>:"Initialize.vi"("Reset (True)"=w303, "VISA resource name"="SR830 #3") -> ("error out"=w307:errorcluster, "VISA resource name out"=w306:refnum<visa-resource-name>)  [unwired: 8 in]
                    n76 = call <instrlib>:"Configure Input Signal.vi"("Input Notch Filter (0: None)"="SR830 #3 Input\nNotch Filter", "Input Shield Grounding (0: Float)"="SR830 #3 Input \nShield Grounding", "error in (no error)"=w307, "Input Coupling (0: AC)"="SR830 #3\nInput Coupling", "Input Connection (0: Single-Ended Voltage)"="SR830 #3 Input Connection", "VISA resource name"=w306) -> ("error out"=w309:errorcluster, "VISA resource name out"=w308:refnum<visa-resource-name>)  [unwired: 4 in]
                    n77 = call <instrlib>:"Configure Trigger.vi"("error in (no error)"=w309, "Trigger Source (0: Internal)"="SR830 #3 Trigger Source", "VISA resource name"=w308) -> ("error out"=w311:errorcluster, "VISA resource name out"=w310:refnum<visa-resource-name>)  [unwired: 7 in]
                    n78 = call <instrlib>:"Configure Reference.vi"("VISA resource name"=w310, "Auto Phase (T: Enabled)"="SR830 #3 \nAuto Phase", "Manual Phase (0 Degree)"="SR830 #3 Manual \nPhase", "Reference Source (1: Internal)"="SR830 #3 Reference Source", "Sine Output Amplitude (1 V)"="Output Amp #3", "Detection Harmonic Number (1)"="SR830 #3 Detection Harm. Num.", "error in (no error)"=w311, "Internal Reference Frequency (1000 Hz)"="SR830 #3 Internal \nReference Frequency", "External Reference Trigger (0: Sine Zero Crossing)"="External Reference Trigger (0: Sine Zero Crossing)  2") -> ("VISA resource name out"=w313:refnum<visa-resource-name>, "error out"=w312:errorcluster)  [unwired: 5 in]
                    n79 = Bundle(cluster=w294, "Voltage Output"="Output Amp #3") -> (w292:T7)  [unwired: 2 in]
                    n80 = Bundle(cluster=w297, "Sensitivity"="SR830 #3 Initial\nSensitivity") -> (w296:T8)  [unwired: 2 in]
                    n81 = call <instrlib>:"Configure Filter.vi"("Enable Sync Filter (F: Disable)"="SR830 #3\nSync Filter", "error in (no error)"=w312, "Low Pass Filter Slope (1: 12dB/oct)"="SR830 #3 Low\nPass Filter Slope", "Time Constant (8: 100ms)"="SR830 #3 \nTime Constant", "VISA resource name"=w313) -> ("error out"=w325:errorcluster, "VISA resource name out"=w324:refnum<visa-resource-name>)  [unwired: 5 in]
                    n82 = call <instrlib>:"Configure Sensitivity and Reserve.vi"("error in (no error)"=w325, "Sensitivity (-1: Auto gain)"="SR830 #3 Initial\nSensitivity", "Dynamic Reserve (-1: Auto Reserve)"="SR830 #3 \nDynamic Reserve", "VISA resource name"=w324) -> ("error out"=w327:errorcluster, "VISA resource name out"=w326:refnum<visa-resource-name>)  [unwired: 6 in]
                    n83 = Bundle(cluster=w302, "Initialised?"=w289) -> (w301:T4)  [unwired: 2 in]
                    n84 = Bundle("VISA resource name out"=w326, "error out"=w327) -> (w298:T3)  [unwired: 1 in]
                    n85 = Bundle(cluster=w300, "Reference & Errors"=w298) -> (w299:T6)  [unwired: 2 in]
                  }
                }
              }
            }
            n86 = Build Array(w83, w82, w84) -> (w85:bool[])
            n87 = Or Array Elements(Boolean array=w85) -> (logical OR=w81:bool)
          }
          frame #1 {
            # "PPMS Initialisation\nNote: HAS to be initalised"
            n88 = flat-sequence {
              tunnel: w338 -> [w347]
              tunnel: [w346] -> w336
              tunnel: [w345] -> w335
              tunnel: [w344] -> w334
              tunnel: [w343] -> _
              tunnel: w331 -> [w343]
              tunnel: [w369] -> w337
              tunnel: w336 -> [w369]
              tunnel: w335 -> [w361]
              tunnel: w334 -> [w360]
              tunnel: [w359] -> w333
              tunnel: [w358] -> w332
              frame #0 {
                n89 = case shown="False" w347 {
                  selector: w347 -> [_ w357]
                  tunnel: [TRUE ("WaitForChamber") w357] -> w346
                  tunnel: [w349 w355] -> w345
                  tunnel: [w348 w356] -> w344
                  tunnel: w343 -> [_ w354]
                  frame False {
                    w351 = 0 items=["PPMS", "VersaLab", "DynaCool", "SVSM"] ("Instrument Type")
                    n90 = call "OpenQDInstrument.vi"("Remote"="Remote", "IP Address"="127.0.0.1", "Instrument Type"=w351) -> ("error out"=w349:errorcluster, "Instrument Ref"=w348:refnum<k24>)  [unwired: 5 in]
                  }
                  frame True {
                    n91 = Unbundle(w354) -> ("Instrument Ref Out"=w356:refnum<k24>, "error out"=w355:errorcluster)
                  }
                }
              }
              frame #1 {
                n92 = call "WaitFor.vi"("Wait For Chamber"=TRUE ("WaitForChamber"), "Wait For Position"=FALSE ("WaitForPosition"), "Wait For Field"=FALSE ("WaitForField"), "Wait For Temperature"=FALSE ("WaitForTemperature"), "error in (no error)"=w361, "Instrument Ref In"=w360) -> ("error out"=w368:errorcluster, "Instrument Ref Out"=w367:refnum<k24>)  [unwired: 4 in]
                n93 = call "GetChamber.vi"("error in (no error)"=w368, "Instrument Ref In"=w367) -> ("Chamber\nStatus"=→"PPMS Chamber Status":i32, "error out"=w358:errorcluster, "Instrument Ref Out"=w359:refnum<k24>)  [unwired: 2 in, 1 out]
              }
            }
            n94 = Bundle(cluster=w331, "Instrument Ref Out"=w333, "error out"=w332) -> (w330:T2)
          }
        }
      }
      frame #1 {
        # "Measurements"
        n95 = flat-sequence {
          tunnel: w372 -> [w379]
          tunnel: [w378] -> w371
          tunnel: [w390] -> w375
          tunnel: w373 -> [w389]
          tunnel: w374 -> [w388]
          frame #0 {
            # "PPMS Measurements"
            n96 = Unbundle(w379) -> ("Instrument Ref Out"=w383:refnum<k24>, "error out"=w382:errorcluster)
            n97 = call "GetTemperature.vi"("error in (no error)"=w382, "Instrument Ref In"=w383) -> ("Temperature"=→"Temperature":dbl, "error out"=w386:errorcluster, "Instrument Ref Out"=w387:refnum<k24>)  [unwired: 3 in, 2 out]
            n98 = call "GetField.vi"("error in (no error)"=w386, "Instrument Ref In"=w387) -> ("Field"=→"Field":dbl, "error out"=w380:errorcluster, "Instrument Ref Out"=w381:refnum<k24>)  [unwired: 3 in, 2 out]
            n99 = Bundle(cluster=w379, "Instrument Ref Out"=w381, "error out"=w380) -> (w378:T2)
          }
          frame #1 {
            # "SR830-Lockin-Amplifier Measurements"
            n100 = stacked-sequence {
              seq-local: [_ w413 _] -> [_ _ w432]
              seq-local: [w394 _ _] -> [_ w411 _]
              tunnel: w389 -> [w393 w414 w434]
              tunnel: w388 -> [w395 _ _]
              tunnel: [_ _ w429] -> w390
              frame #0 {
                n101 = Unbundle(w395) -> ("Reference & Errors"=w391:T3)  [unwired: 2 out]
                n102 = Unbundle(w393) -> ("Initialised?"=w396:bool)  [unwired: 2 out]
                n103 = case shown="True" w396 {
                  tunnel: [w397 w404] -> w392
                  tunnel: w391 -> [w397 w403]
                  frame False {
                  }
                  frame True {
                    n104 = Unbundle(w403) -> ("VISA resource name out"=w409:refnum<visa-resource-name>, "error out"=w408:errorcluster)
                    n105 = call-poly <instrlib>:"Read.vi"("error in (no error)"=w408, "VISA resource name"=w409) -> ("error out"=w406:errorcluster, "Parameter Values"=w407:T10, "VISA resource name out"=w405:refnum<visa-resource-name>)  [unwired: 7 in]
                    n106 = Bundle("VISA resource name out"=w405, "error out"=w406) -> (w404:T3)  [unwired: 1 in]
                    n107 = Unbundle(w407) -> ("X-Value"=→"X-Value":dbl, "Y-Value"=→"Y-Value":dbl, "R-Value"=→"R-Value":dbl, "Theta-Value"=→"Theta-Value":dbl, "Reference Frequency"=→"Reference Freq":dbl)  [unwired: 6 out]
                  }
                }
                n108 = Bundle(cluster=w395, "Reference & Errors"=w392) -> (w394:T6)  [unwired: 2 in]
              }
              frame #1 {
                n109 = Unbundle(w411) -> ("Reference & Errors"=w412:T3)  [unwired: 2 out]
                n110 = Unbundle(w414) -> ("Initialised?"=w415:bool)  [unwired: 2 out]
                n111 = case shown="True" w415 {
                  tunnel: w412 -> [w416 w428]
                  tunnel: [w416 w422] -> w410
                  frame False {
                  }
                  frame True {
                    n112 = Unbundle(w428) -> ("VISA resource name out"=w427:refnum<visa-resource-name>, "error out"=w426:errorcluster)
                    n113 = call-poly <instrlib>:"Read.vi"("error in (no error)"=w426, "VISA resource name"=w427) -> ("error out"=w423:errorcluster, "Parameter Values"=w425:T10, "VISA resource name out"=w424:refnum<visa-resource-name>)  [unwired: 7 in]
                    n114 = Unbundle(w425) -> ("X-Value"=→"X-Value 2":dbl, "Y-Value"=→"Y-Value 2":dbl, "R-Value"=→"R-Value 2":dbl, "Theta-Value"=→"Theta-Value 2":dbl, "Reference Frequency"=→"Reference Freq 2":dbl)  [unwired: 6 out]
                    n115 = Bundle("VISA resource name out"=w424, "error out"=w423) -> (w422:T3)  [unwired: 1 in]
                  }
                }
                n116 = Bundle(cluster=w411, "Reference & Errors"=w410) -> (w413:T6)  [unwired: 2 in]
              }
              frame #2 {
                n117 = Unbundle(w434) -> ("Initialised?"=w433:bool)  [unwired: 2 out]
                n118 = Unbundle(w432) -> ("Reference & Errors"=w431:T3)  [unwired: 2 out]
                n119 = case shown="True" w433 {
                  tunnel: w431 -> [w435 w447]
                  tunnel: [w435 w441] -> w430
                  frame False {
                  }
                  frame True {
                    n120 = Unbundle(w447) -> ("VISA resource name out"=w446:refnum<visa-resource-name>, "error out"=w445:errorcluster)
                    n121 = call-poly <instrlib>:"Read.vi"("error in (no error)"=w445, "VISA resource name"=w446) -> ("error out"=w442:errorcluster, "Parameter Values"=w444:T10, "VISA resource name out"=w443:refnum<visa-resource-name>)  [unwired: 7 in]
                    n122 = Bundle("VISA resource name out"=w443, "error out"=w442) -> (w441:T3)  [unwired: 1 in]
                    n123 = Unbundle(w444) -> ("X-Value"=→"X-Value 3":dbl, "Y-Value"=→"Y-Value 3":dbl, "R-Value"=→"R-Value 3":dbl, "Theta-Value"=→"Theta-Value 3":dbl, "Reference Frequency"=→"Reference Freq 3":dbl)  [unwired: 6 out]
                  }
                }
                n124 = Bundle(cluster=w432, "Reference & Errors"=w430) -> (w429:T6)  [unwired: 2 in]
              }
            }
          }
        }
      }
      frame #2 {
        # "FileIO"
        n125 = case shown="True" "Record data to file?" {
          tunnel: w454 -> [_ w463]
          tunnel: "Data Save Path:" -> [_ w467]
          tunnel: "<File Name>.dat  (Don't add extension)" -> [_ w466]
          tunnel: w450 -> [_ w465]
          tunnel: w449 -> [w458 w460]
          tunnel: [w458 w459] -> w448
          frame False {
          }
          frame True {
            n126 = Unbundle(w460) -> ("RecordingInProgress"=w464:bool)  [unwired: 3 out]
            n127 = Not(x=w464) -> (.not. x?=w462:bool)
            n128 = Or(x=w463, y=w462) -> (x .or. y?=w461:bool)
            n129 = stacked-sequence {
              seq-local: [w468 _] -> [_ w583]
              tunnel: w461 -> [w470 _]
              tunnel: w467 -> [w473 _]
              tunnel: w466 -> [w472 _]
              tunnel: w465 -> [w471 w579]
              tunnel: w460 -> [w469 _]
              tunnel: [_ w571] -> w459
              frame #0 {
                # "#1 Check if update to SR830 amps. If so, create new file to match headers."
                n130 = case shown="True" w470 {
                  tunnel: w473 -> [_ w519]
                  tunnel: w472 -> [_ w518]
                  tunnel: w471 -> [_ w514]
                  tunnel: w469 -> [w474 w494]
                  tunnel: [w474 w492] -> w468
                  frame False {
                  }
                  frame True {
                    w483 = "\r\n"
                    w499 = "\t"
                    w504 = "V" ("string")
                    # "One of the SR830s is updated or record turned on, and so need a new file / labels"
                    n131 = Unbundle(w494) -> ("RecordingInProgress"=w508:bool, "refnum out"=w507:refnum<file>, "error out"=w506:errorcluster)  [unwired: 1 out]
                    n132 = Unbundle(w514) -> ("Initialised?"=w513:bool, "Initialised?"=w512:bool, "Initialised?"=w511:bool)
                    n133 = case shown="True" w508 {
                      tunnel: w507 -> [_ w521]
                      tunnel: w506 -> [_ w520]
                      frame False {
                      }
                      frame True {
                        # "Need to close old file and create new."
                        n134 = Close File(refnum=w521, error in=w520) -> (error out=w522:errorcluster)  [unwired: 1 out]
                        n135 = call <vilib>:"Simple Error Handler.vi"("error in (no error)"=w522) -> ()  [unwired: 4 in, 5 out]
                      }
                    }
                    n136 = Concatenate Strings(w499, w504, w499, w504, w499, w504, w499, "Degrees" ("string")) -> (w500:string)
                    n137 = call "Initialise_File.vi"("<File Name>.txt (Don't add extension)"=w518, "Data Save Path:"=w519) -> ("error out"=w476:errorcluster, "Actual Save Path"=w491:path, "refnum out"=w478:refnum<file>)  [unwired: 7 in]
                    "Actual Save Path" <- w491
                    n138 = stacked-sequence {
                      seq-local: [w525 _ _] -> [_ w540 _]
                      seq-local: [_ w539 _] -> [_ _ w557]
                      seq-local: [w523 _ _] -> [_ w537 _]
                      seq-local: [_ w535 _] -> [_ _ w553]
                      tunnel: w513 -> [w526 _ _]
                      tunnel: w512 -> [_ w542 _]
                      tunnel: w511 -> [_ _ w558]
                      tunnel: [_ _ w555] -> w510
                      tunnel: w500 -> [w524 w538 w554]
                      tunnel: [_ _ w551] -> w497
                      frame #0 {
                        n139 = case shown="True" w526 {
                          tunnel: [w527 w530] -> w525
                          tunnel: w524 -> [_ w528]
                          tunnel: [w527 w528] -> w523
                          frame False {
                            w527 = "" ("string")
                          }
                          frame True {
                            w529 = "\t"
                            n140 = Concatenate Strings(w529, "X1" ("string"), w529, "Y1" ("string"), w529, "R1" ("string"), w529, "Theta1" ("string")) -> (w530:string)
                          }
                        }
                      }
                      frame #1 {
                        n141 = case shown="True" w542 {
                          tunnel: [w543 w546] -> w541
                          tunnel: w538 -> [_ w544]
                          tunnel: [w543 w544] -> w536
                          frame False {
                            w543 = "" ("string")
                          }
                          frame True {
                            w545 = "\t"
                            n142 = Concatenate Strings(w545, "X2" ("string"), w545, "Y2" ("string"), w545, "R2" ("string"), w545, "Theta2" ("string")) -> (w546:string)
                          }
                        }
                        n143 = Concatenate Strings(w537, w536) -> (w535:string)
                        n144 = Concatenate Strings(w540, w541) -> (w539:string)
                      }
                      frame #2 {
                        n145 = case shown="True" w558 {
                          tunnel: [w559 w562] -> w556
                          tunnel: w554 -> [_ w560]
                          tunnel: [w559 w560] -> w552
                          frame False {
                            w559 = "" ("string")
                          }
                          frame True {
                            w561 = "\t"
                            n146 = Concatenate Strings(w561, "X3" ("string"), w561, "Y3" ("string"), w561, "R3" ("string"), w561, "Theta3" ("string")) -> (w562:string)
                          }
                        }
                        n147 = Concatenate Strings(w553, w552) -> (w551:string)
                        n148 = Concatenate Strings(w557, w556) -> (w555:string)
                      }
                    }
                    n149 = Concatenate Strings("K" ("string"), "\t", "Oe" ("string")) -> (w498:string)
                    n150 = Concatenate Strings("Temperature" ("string"), "\t", "Field" ("string")) -> (w509:string)
                    n151 = Concatenate Strings(w509, w510) -> (w496:string)
                    n152 = Concatenate Strings(w498, w497) -> (w495:string)
                    n153 = Get Date/Time String(date format (0)=enum16{"short", "long", "abbreviated"}."short", want seconds? (F)=TRUE) -> (date string=w485:string, time string=w484:string)  [unwired: 1 in]
                    n154 = Concatenate Strings("Time" ("string"), "\t", w485, " " ("string"), w484) -> (w481:string)
                    n155 = Concatenate Strings("File Notes:", w483, w481, w483, "[Data]" ("string"), w483, w496, w483, w495, w483) -> (w479:string)
                    n156 = Write to Text File(file (use dialog)=w478, text=w479, error in=w476) -> (refnum out=w477:refnum<file>, error out=w475:errorcluster)  [unwired: 1 in, 1 out]
                    n157 = Bundle(cluster=w494, "RecordingInProgress"=TRUE, "refnum out"=w477, "error out"=w475, "Actual Save Path"=w491) -> (w492:T5)
                  }
                }
              }
              frame #1 {
                # "#2 Write values to file."
                n158 = Unbundle(w579) -> ("Initialised?"=w578:bool, "Initialised?"=w577:bool, "Initialised?"=w576:bool)
                n159 = Unbundle(w583) -> ("refnum out"=w585:refnum<file>, "error out"=w584:errorcluster)  [unwired: 2 out]
                n160 = stacked-sequence {
                  seq-local: [w586 _ _] -> [_ w603 _]
                  seq-local: [_ w601 _] -> [_ _ w620]
                  tunnel: w578 -> [w588 _ _]
                  tunnel: w577 -> [_ w605 _]
                  tunnel: w576 -> [_ _ w622]
                  tunnel: "Data Format String" -> [w587 w604 w621]
                  tunnel: [_ _ w619] -> w569
                  frame #0 {
                    n161 = case shown="True" w588 {
                      tunnel: w587 -> [_ w591]
                      tunnel: ["" ("format string") w590] -> w586
                      frame False {
                      }
                      frame True {
                        w592 = "\t"
                        n162 = local read "Theta-Value"() -> (w600:dbl)
                        n163 = local read "X-Value"() -> (w597:dbl)
                        n164 = local read "Y-Value"() -> (w598:dbl)
                        n165 = local read "R-Value"() -> (w599:dbl)
                        n166 = Format Into String(format string=w591, w597) -> (resulting string=w593:string)  [unwired: 2 in, 1 out]
                        n167 = Format Into String(format string=w591, w598) -> (resulting string=w594:string)  [unwired: 2 in, 1 out]
                        n168 = Format Into String(format string=w591, w599) -> (resulting string=w595:string)  [unwired: 2 in, 1 out]
                        n169 = Format Into String(format string=w591, w600) -> (resulting string=w596:string)  [unwired: 2 in, 1 out]
                        n170 = Concatenate Strings(w592, w593, w592, w594, w592, w595, w592, w596) -> (w590:string)
                      }
                    }
                  }
                  frame #1 {
                    n171 = case shown="True" w605 {
                      tunnel: w604 -> [_ w608]
                      tunnel: ["" ("format string") w607] -> w602
                      frame False {
                      }
                      frame True {
                        w609 = "\t"
                        n172 = local read "Theta-Value 2"() -> (w617:dbl)
                        n173 = local read "X-Value 2"() -> (w614:dbl)
                        n174 = local read "Y-Value 2"() -> (w615:dbl)
                        n175 = local read "R-Value 2"() -> (w616:dbl)
                        n176 = Format Into String(format string=w608, w614) -> (resulting string=w610:string)  [unwired: 2 in, 1 out]
                        n177 = Format Into String(format string=w608, w615) -> (resulting string=w611:string)  [unwired: 2 in, 1 out]
                        n178 = Format Into String(format string=w608, w616) -> (resulting string=w612:string)  [unwired: 2 in, 1 out]
                        n179 = Format Into String(format string=w608, w617) -> (resulting string=w613:string)  [unwired: 2 in, 1 out]
                        n180 = Concatenate Strings(w609, w610, w609, w611, w609, w612, w609, w613) -> (w607:string)
                      }
                    }
                    n181 = Concatenate Strings(w603, w602) -> (w601:string)
                  }
                  frame #2 {
                    n182 = case shown="True" w622 {
                      tunnel: w621 -> [_ w625]
                      tunnel: ["" ("format string") w624] -> w618
                      frame False {
                      }
                      frame True {
                        w626 = "\t"
                        n183 = local read "Theta-Value 3"() -> (w634:dbl)
                        n184 = local read "X-Value 3"() -> (w631:dbl)
                        n185 = local read "Y-Value 3"() -> (w632:dbl)
                        n186 = local read "R-Value 3"() -> (w633:dbl)
                        n187 = Format Into String(format string=w625, w631) -> (resulting string=w627:string)  [unwired: 2 in, 1 out]
                        n188 = Format Into String(format string=w625, w632) -> (resulting string=w628:string)  [unwired: 2 in, 1 out]
                        n189 = Format Into String(format string=w625, w633) -> (resulting string=w629:string)  [unwired: 2 in, 1 out]
                        n190 = Format Into String(format string=w625, w634) -> (resulting string=w630:string)  [unwired: 2 in, 1 out]
                        n191 = Concatenate Strings(w626, w627, w626, w628, w626, w629, w626, w630) -> (w624:string)
                      }
                    }
                    n192 = Concatenate Strings(w620, w618) -> (w619:string)
                  }
                }
                n193 = local read "Temperature"() -> (w575:dbl)
                n194 = local read "Field"() -> (w574:dbl)
                n195 = Format Into String(format string="Data Format String", w575) -> (resulting string=w572:string)  [unwired: 2 in, 1 out]
                n196 = Format Into String(format string="Data Format String", w574) -> (resulting string=w573:string)  [unwired: 2 in, 1 out]
                n197 = Concatenate Strings(w572, "\t", w573) -> (w570:string)
                n198 = Concatenate Strings(w570, w569) -> (w568:string)
                n199 = Write to Text File(file (use dialog)=w585, text=w568, error in=w584) -> (refnum out=w582:refnum<file>, error out=w581:errorcluster)  [unwired: 1 in, 1 out]
                n200 = Bundle(cluster=w583, "refnum out"=w582, "error out"=w581) -> (w571:T5)  [unwired: 2 in]
              }
            }
          }
        }
      }
      frame #3 {
        # "SR830 Source Signal Change - Source Input Voltage Adjustment"
        n201 = stacked-sequence {
          seq-local: [w647 _ _] -> [_ w677 _]
          seq-local: [_ w673 _] -> [_ _ w703]
          seq-local: [w641 _ _] -> [_ w671 _]
          seq-local: [_ w670 _] -> [_ _ w700]
          tunnel: w639 -> [w642 _ _]
          tunnel: w638 -> [w646 w676 w706]
          tunnel: w637 -> [w648 _ _]
          tunnel: [_ _ w702] -> w636
          tunnel: [_ _ w699] -> w635
          frame #0 {
            n202 = Unbundle(w646) -> ("Initialised?"=w645:bool)  [unwired: 2 out]
            n203 = Unbundle(w642) -> ("Voltage Output"=w644:dbl)  [unwired: 2 out]
            n204 = local read "Output Amp #1"() -> (w643:dbl)
            n205 = Not Equal?(x=w643, y=w644) -> (x != y?=w649:bool)
            n206 = And(x=w645, y=w649) -> (x .and. y?=w650:bool)
            n207 = case shown="True" w650 {
              tunnel: w648 -> [w652 w663]
              tunnel: [w652 w662] -> w647
              tunnel: w643 -> [_ w654]
              tunnel: w642 -> [w651 w655]
              tunnel: [w651 w653] -> w641
              frame False {
              }
              frame True {
                n208 = local read "SR830 #1 Manual \nPhase"() -> (w661:dbl)
                n209 = local read "SR830 #1 \nAuto Phase"() -> (w660:bool)
                n210 = local read "SR830 #1 Detection Harm. Num."() -> (w658:dbl)
                n211 = local read "External Reference Trigger (0: Sine Zero Crossing)"() -> (w656:u16)
                n212 = local read "SR830 #1 Reference Source"() -> (w659:u16)
                n213 = local read "SR830 #1 Internal \nReference Frequency"() -> (w657:dbl)
                n214 = Unbundle(w663) -> ("Reference & Errors"=w665:T3)  [unwired: 2 out]
                n215 = Unbundle(w665) -> ("VISA resource name out"=w669:refnum<visa-resource-name>, "error out"=w668:errorcluster)
                n216 = Bundle(cluster=w655, "Voltage Output"=w654) -> (w653:T7)  [unwired: 2 in]
                n217 = call <instrlib>:"Configure Reference.vi"("VISA resource name"=w669, "Auto Phase (T: Enabled)"=w660, "Manual Phase (0 Degree)"=w661, "Reference Source (1: Internal)"=w659, "Sine Output Amplitude (1 V)"=w654, "Detection Harmonic Number (1)"=w658, "error in (no error)"=w668, "Internal Reference Frequency (1000 Hz)"=w657, "External Reference Trigger (0: Sine Zero Crossing)"=w656) -> ("VISA resource name out"=w667:refnum<visa-resource-name>, "error out"=w666:errorcluster)  [unwired: 5 in]
                n218 = Bundle(cluster=w665, "VISA resource name out"=w667, "error out"=w666) -> (w664:T3)
                n219 = Bundle(cluster=w663, "Reference & Errors"=w664) -> (w662:T6)  [unwired: 2 in]
              }
            }
          }
          frame #1 {
            n220 = Unbundle(w676) -> ("Initialised?"=w675:bool)  [unwired: 2 out]
            n221 = Unbundle(w671) -> ("Voltage Output"=w674:dbl)  [unwired: 2 out]
            n222 = local read "Output Amp #2"() -> (w672:dbl)
            n223 = Not Equal?(x=w672, y=w674) -> (x != y?=w678:bool)
            n224 = And(x=w675, y=w678) -> (x .and. y?=w679:bool)
            n225 = case shown="True" w679 {
              tunnel: w677 -> [w681 w691]
              tunnel: [w681 w692] -> w673
              tunnel: w672 -> [_ w683]
              tunnel: w671 -> [w680 w684]
              tunnel: [w680 w682] -> w670
              frame False {
              }
              frame True {
                n226 = local read "SR830 #2 Internal \nReference Frequency"() -> (w690:dbl)
                n227 = local read "External Reference Trigger #2 (0: Sine Zero Crossing)"() -> (w689:u16)
                n228 = local read "SR830 #2 Detection Harm. Num."() -> (w688:dbl)
                n229 = local read "SR830 #2 Reference Source"() -> (w687:u16)
                n230 = local read "SR830 #2 \nAuto Phase"() -> (w686:bool)
                n231 = local read "SR830 #2 Manual \nPhase"() -> (w685:dbl)
                n232 = Unbundle(w691) -> ("Reference & Errors"=w694:T3)  [unwired: 2 out]
                n233 = Unbundle(w694) -> ("VISA resource name out"=w698:refnum<visa-resource-name>, "error out"=w697:errorcluster)
                n234 = Bundle(cluster=w684, "Voltage Output"=w683) -> (w682:T7)  [unwired: 2 in]
                n235 = call <instrlib>:"Configure Reference.vi"("VISA resource name"=w698, "Auto Phase (T: Enabled)"=w686, "Manual Phase (0 Degree)"=w685, "Reference Source (1: Internal)"=w687, "Sine Output Amplitude (1 V)"=w683, "Detection Harmonic Number (1)"=w688, "error in (no error)"=w697, "Internal Reference Frequency (1000 Hz)"=w690, "External Reference Trigger (0: Sine Zero Crossing)"=w689) -> ("VISA resource name out"=w696:refnum<visa-resource-name>, "error out"=w695:errorcluster)  [unwired: 5 in]
                n236 = Bundle(cluster=w694, "VISA resource name out"=w696, "error out"=w695) -> (w693:T3)
                n237 = Bundle(cluster=w691, "Reference & Errors"=w693) -> (w692:T6)  [unwired: 2 in]
              }
            }
          }
          frame #2 {
            n238 = Unbundle(w706) -> ("Initialised?"=w705:bool)  [unwired: 2 out]
            n239 = Unbundle(w700) -> ("Voltage Output"=w704:dbl)  [unwired: 2 out]
            n240 = local read "Output Amp #3"() -> (w701:dbl)
            n241 = Not Equal?(x=w701, y=w704) -> (x != y?=w707:bool)
            n242 = And(x=w705, y=w707) -> (x .and. y?=w708:bool)
            n243 = case shown="True" w708 {
              tunnel: w703 -> [w710 w721]
              tunnel: [w710 w720] -> w702
              tunnel: w701 -> [_ w712]
              tunnel: w700 -> [w709 w713]
              tunnel: [w709 w711] -> w699
              frame False {
              }
              frame True {
                n244 = local read "SR830 #3 Manual \nPhase"() -> (w716:dbl)
                n245 = local read "SR830 #3 \nAuto Phase"() -> (w717:bool)
                n246 = local read "SR830 #3 Internal \nReference Frequency"() -> (w714:dbl)
                n247 = local read "SR830 #3 Detection Harm. Num."() -> (w715:dbl)
                n248 = local read "External Reference Trigger (0: Sine Zero Crossing)  2"() -> (w719:u16)
                n249 = local read "SR830 #3 Reference Source"() -> (w718:u16)
                n250 = Unbundle(w721) -> ("Reference & Errors"=w723:T3)  [unwired: 2 out]
                n251 = Bundle(cluster=w713, "Voltage Output"=w712) -> (w711:T7)  [unwired: 2 in]
                n252 = Unbundle(w723) -> ("VISA resource name out"=w727:refnum<visa-resource-name>, "error out"=w726:errorcluster)
                n253 = call <instrlib>:"Configure Reference.vi"("VISA resource name"=w727, "Auto Phase (T: Enabled)"=w717, "Manual Phase (0 Degree)"=w716, "Reference Source (1: Internal)"=w718, "Sine Output Amplitude (1 V)"=w712, "Detection Harmonic Number (1)"=w715, "error in (no error)"=w726, "Internal Reference Frequency (1000 Hz)"=w714, "External Reference Trigger (0: Sine Zero Crossing)"=w719) -> ("VISA resource name out"=w725:refnum<visa-resource-name>, "error out"=w724:errorcluster)  [unwired: 5 in]
                n254 = Bundle(cluster=w723, "VISA resource name out"=w725, "error out"=w724) -> (w722:T3)
                n255 = Bundle(cluster=w721, "Reference & Errors"=w722) -> (w720:T6)  [unwired: 2 in]
              }
            }
          }
        }
      }
      frame #4 {
        # "SR830 Custom auto adjustment sensitivity"
        n256 = stacked-sequence {
          seq-local: [_ w797 _] -> [_ _ w857]
          seq-local: [w742 _ _] -> [_ w796 _]
          seq-local: [w741 _ _] -> [_ w801 _]
          seq-local: [_ w798 _] -> [_ _ w852]
          tunnel: w739 -> [w745 _ _]
          tunnel: [_ _ w853] -> w738
          tunnel: [_ _ w856] -> w737
          tunnel: w736 -> [w744 w800 w855]
          tunnel: w729 -> [w740 _ _]
          frame #0 {
            n257 = Unbundle(w744) -> ("Initialised?"=w743:bool)  [unwired: 2 out]
            n258 = case shown="True" w743 {
              tunnel: w745 -> [w747 w756]
              tunnel: [w747 w755] -> w742
              tunnel: [w746 w752] -> w741
              tunnel: w740 -> [w746 w749]
              frame False {
              }
              frame True {
                n259 = Unbundle(w756) -> ("Sensitivity"=w759:i16)  [unwired: 2 out]
                n260 = call "SR830_sensitivity_de-enumerator.vi"("Sensitivity (Initial Value)"=w759) -> ("Sensitivity (nV/fA)"=w757:dbl)  [unwired: 10 in]
                n261 = local read "R-Value"() -> (w748:dbl)
                n262 = Divide(x=w757, y=1000000000.0) -> (x/y=w760:dbl)
                n263 = Absolute Value(x=w748) -> (abs(x)=w750:dbl)
                n264 = Multiply(x=w760, y=0.9) -> (x*y=w768:dbl)
                n265 = Multiply(x=w760, y=0.25) -> (x*y=w767:dbl)
                n266 = Less?(x=w750, y=w767) -> (x < y?=w764:bool)
                "Sense Under" <- w764
                n267 = Greater?(x=w750, y=w768) -> (0:w763:bool)
                "Sense Over" <- w763
                n268 = Or(x=w764, y=w763) -> (x .or. y?=w762:bool)
                n269 = case shown="True" w764 {
                  tunnel: w759 -> [w792 w795]
                  tunnel: [w792 w793] -> w766
                  frame False {
                  }
                  frame True {
                    n270 = Subtract(x=w795, y=i16 1) -> (x-y=w793:i16)
                  }
                }
                n271 = local read "SR830 #1 \nDynamic Reserve"() -> (w758:i16)
                n272 = case shown="True" w763 {
                  tunnel: w766 -> [w788 w791]
                  tunnel: [w788 w789] -> w765
                  frame False {
                  }
                  frame True {
                    n273 = Add(x=w791, y=i16 1) -> (x+y=w789:i16)
                  }
                }
                n274 = Unbundle(w749) -> ("Reference & Errors"=w754:T3)  [unwired: 2 out]
                n275 = case shown="True" w762 {
                  tunnel: w765 -> [w772 w780]
                  tunnel: [w772 w780] -> w751
                  tunnel: w758 -> [_ w787]
                  tunnel: w754 -> [w771 w775]
                  tunnel: [w771 w783] -> w753
                  frame False {
                  }
                  frame True {
                    n276 = local read "SR830 #1 \nTime Constant"() -> (w779:u16)
                    n277 = call "SR830_time_constant_de-enumerator.vi"("Time Constant (8: 100ms)"=w779) -> ("Time Constant (us)"=w778:dbl)  [unwired: 10 in]
                    n278 = Divide(x=w778, y=1000000.0) -> (x/y=w776:dbl)
                    n279 = Unbundle(w775) -> ("VISA resource name out"=w774:refnum<visa-resource-name>, "error out"=w773:errorcluster)
                    n280 = call <instrlib>:"Configure Sensitivity and Reserve.vi"("error in (no error)"=w773, "Sensitivity (-1: Auto gain)"=w780, "Dynamic Reserve (-1: Auto Reserve)"=w787, "VISA resource name"=w774) -> ("error out"=w782:errorcluster, "VISA resource name out"=w784:refnum<visa-resource-name>)  [unwired: 6 in]
                    n281 = Multiply(x=w776, y=3.0) -> (x*y=w786:dbl)
                    n282 = call "Time Delay"("error in (no error)"=w782, "Delay Time (s)"=w786) -> ("error out"=w781:errorcluster)  [unwired: 9 in]
                    n283 = Bundle("VISA resource name out"=w784, "error out"=w781) -> (w783:T3)  [unwired: 1 in]
                  }
                }
                n284 = Bundle(cluster=w756, "Sensitivity"=w751) -> (w755:T8)  [unwired: 2 in]
                n285 = Bundle(cluster=w749, "Reference & Errors"=w753) -> (w752:T6)  [unwired: 2 in]
              }
            }
          }
          frame #1 {
            n286 = Unbundle(w800) -> ("Initialised?"=w799:bool)  [unwired: 2 out]
            n287 = case shown="True" w799 {
              tunnel: w796 -> [w802 w815]
              tunnel: [w802 w814] -> w797
              tunnel: w801 -> [w803 w812]
              tunnel: [w803 w811] -> w798
              frame False {
              }
              frame True {
                n288 = Unbundle(w815) -> ("Sensitivity"=w807:i16)  [unwired: 2 out]
                n289 = local read "R-Value 2"() -> (w804:dbl)
                n290 = call "SR830_sensitivity_de-enumerator.vi"("Sensitivity (Initial Value)"=w807) -> ("Sensitivity (nV/fA)"=w810:dbl)  [unwired: 10 in]
                n291 = Divide(x=w810, y=1000000000.0) -> (x/y=w816:dbl)
                n292 = Absolute Value(x=w804) -> (abs(x)=w806:dbl)
                n293 = Multiply(x=w816, y=0.9) -> (x*y=w824:dbl)
                n294 = Multiply(x=w816, y=0.25) -> (x*y=w823:dbl)
                n295 = Less?(x=w806, y=w823) -> (x < y?=w820:bool)
                "Sense\nUnder 2" <- w820
                n296 = Greater?(x=w806, y=w824) -> (0:w819:bool)
                "Sense\nOver 2" <- w819
                n297 = case shown="True" w820 {
                  tunnel: [w848 w850] -> w822
                  tunnel: w807 -> [w848 w849]
                  frame False {
                  }
                  frame True {
                    n298 = Subtract(x=w849, y=i16 1) -> (x-y=w850:i16)
                  }
                }
                n299 = Or(x=w820, y=w819) -> (x .or. y?=w818:bool)
                n300 = Unbundle(w812) -> ("Reference & Errors"=w813:T3)  [unwired: 2 out]
                n301 = local read "SR830 #2 \nDynamic Reserve"() -> (w809:i16)
                n302 = case shown="True" w819 {
                  tunnel: w822 -> [w844 w847]
                  tunnel: [w844 w845] -> w821
                  frame False {
                  }
                  frame True {
                    n303 = Add(x=w847, y=i16 1) -> (x+y=w845:i16)
                  }
                }
                n304 = case shown="True" w818 {
                  tunnel: w821 -> [w828 w843]
                  tunnel: [w828 w843] -> w808
                  tunnel: w813 -> [w827 w831]
                  tunnel: [w827 w838] -> w805
                  tunnel: w809 -> [_ w836]
                  frame False {
                  }
                  frame True {
                    n305 = local read "SR830 #2 \nTime Constant"() -> (w833:u16)
                    n306 = call "SR830_time_constant_de-enumerator.vi"("Time Constant (8: 100ms)"=w833) -> ("Time Constant (us)"=w835:dbl)  [unwired: 10 in]
                    n307 = Unbundle(w831) -> ("VISA resource name out"=w830:refnum<visa-resource-name>, "error out"=w829:errorcluster)
                    n308 = Divide(x=w835, y=1000000.0) -> (x/y=w832:dbl)
                    n309 = call <instrlib>:"Configure Sensitivity and Reserve.vi"("error in (no error)"=w829, "Sensitivity (-1: Auto gain)"=w843, "Dynamic Reserve (-1: Auto Reserve)"=w836, "VISA resource name"=w830) -> ("error out"=w839:errorcluster, "VISA resource name out"=w840:refnum<visa-resource-name>)  [unwired: 6 in]
                    n310 = Multiply(x=w832, y=3.0) -> (x*y=w842:dbl)
                    n311 = call "Time Delay2"("error in (no error)"=w839, "Delay Time (s)"=w842) -> ("error out"=w837:errorcluster)  [unwired: 9 in]
                    n312 = Bundle("VISA resource name out"=w840, "error out"=w837) -> (w838:T3)  [unwired: 1 in]
                  }
                }
                n313 = Bundle(cluster=w815, "Sensitivity"=w808) -> (w814:T8)  [unwired: 2 in]
                n314 = Bundle(cluster=w812, "Reference & Errors"=w805) -> (w811:T6)  [unwired: 2 in]
              }
            }
          }
          frame #2 {
            n315 = Unbundle(w855) -> ("Initialised?"=w854:bool)  [unwired: 2 out]
            n316 = case shown="True" w854 {
              tunnel: w857 -> [w859 w864]
              tunnel: [w859 w870] -> w853
              tunnel: [w858 w868] -> w856
              tunnel: w852 -> [w858 w863]
              frame False {
              }
              frame True {
                n317 = Unbundle(w864) -> ("Sensitivity"=w862:i16)  [unwired: 2 out]
                n318 = local read "R-Value 3"() -> (w860:dbl)
                n319 = Unbundle(w863) -> ("Reference & Errors"=w869:T3)  [unwired: 2 out]
                n320 = call "SR830_sensitivity_de-enumerator.vi"("Sensitivity (Initial Value)"=w862) -> ("Sensitivity (nV/fA)"=w866:dbl)  [unwired: 10 in]
                n321 = Divide(x=w866, y=1000000000.0) -> (x/y=w871:dbl)
                n322 = Absolute Value(x=w860) -> (abs(x)=w861:dbl)
                n323 = Multiply(x=w871, y=0.9) -> (x*y=w879:dbl)
                n324 = Multiply(x=w871, y=0.25) -> (x*y=w878:dbl)
                n325 = Less?(x=w861, y=w878) -> (x < y?=w875:bool)
                "Sense\nUnder 3" <- w875
                n326 = Greater?(x=w861, y=w879) -> (0:w874:bool)
                "Sense\nOver 3" <- w874
                n327 = case shown="True" w875 {
                  tunnel: [w903 w905] -> w877
                  tunnel: w862 -> [w903 w904]
                  frame False {
                  }
                  frame True {
                    n328 = Subtract(x=w904, y=i16 1) -> (x-y=w905:i16)
                  }
                }
                n329 = Or(x=w875, y=w874) -> (x .or. y?=w873:bool)
                n330 = local read "SR830 #3 \nDynamic Reserve"() -> (w867:i16)
                n331 = case shown="True" w874 {
                  tunnel: w877 -> [w899 w902]
                  tunnel: [w899 w900] -> w876
                  frame False {
                  }
                  frame True {
                    n332 = Add(x=w902, y=i16 1) -> (x+y=w900:i16)
                  }
                }
                n333 = case shown="True" w873 {
                  tunnel: w876 -> [w883 w898]
                  tunnel: [w883 w898] -> w865
                  tunnel: w869 -> [w882 w886]
                  tunnel: [w882 w892] -> _
                  tunnel: w867 -> [_ w891]
                  frame False {
                  }
                  frame True {
                    n334 = local read "SR830 #3 \nTime Constant"() -> (w888:u16)
                    n335 = call "SR830_time_constant_de-enumerator.vi"("Time Constant (8: 100ms)"=w888) -> ("Time Constant (us)"=w890:dbl)  [unwired: 10 in]
                    n336 = Unbundle(w886) -> ("VISA resource name out"=w885:refnum<visa-resource-name>, "error out"=w884:errorcluster)
                    n337 = Divide(x=w890, y=1000000.0) -> (x/y=w887:dbl)
                    n338 = call <instrlib>:"Configure Sensitivity and Reserve.vi"("error in (no error)"=w884, "Sensitivity (-1: Auto gain)"=w898, "Dynamic Reserve (-1: Auto Reserve)"=w891, "VISA resource name"=w885) -> ("error out"=w897:errorcluster, "VISA resource name out"=w893:refnum<visa-resource-name>)  [unwired: 6 in]
                    n339 = Multiply(x=w887, y=3.0) -> (x*y=w896:dbl)
                    n340 = call "Time Delay3"("error in (no error)"=w897, "Delay Time (s)"=w896) -> ("error out"=w894:errorcluster)  [unwired: 9 in]
                    n341 = Bundle("VISA resource name out"=w893, "error out"=w894) -> (w892:T3)  [unwired: 1 in]
                  }
                }
                n342 = Bundle(cluster=w864, "Sensitivity"=w865) -> (w870:T8)  [unwired: 2 in]
                n343 = Bundle(cluster=w863) -> (w868:T6)  [unwired: 3 in]
              }
            }
          }
        }
        n344 = Unbundle(w738) -> ("Sensitivity"=w734:i16, "Sensitivity"=w733:i16, "Sensitivity"=w731:i16)
        n345 = call "SR830_sensitivity_de-enumerator.vi"("Sensitivity (Initial Value)"=w734) -> ("Sensitivity (nV/fA)"=→"SR830 #3 Sensitivity":dbl)  [unwired: 10 in]
        n346 = call "SR830_sensitivity_de-enumerator.vi"("Sensitivity (Initial Value)"=w731) -> ("Sensitivity (nV/fA)"=→"SR830 #3 Sensitivity 3":dbl)  [unwired: 10 in]
        n347 = call "SR830_sensitivity_de-enumerator.vi"("Sensitivity (Initial Value)"=w733) -> ("Sensitivity (nV/fA)"=→"SR830 #3 Sensitivity 2":dbl)  [unwired: 10 in]
      }
    }
    n348 = Wait (ms)(milliseconds to wait="Loop Timing (ms)") -> ()  [unwired: 1 out]
    "Device Intialization" <- w62
    "PPMS Initialisation" <- w46
  }
  n349 = local write "program_stop"(FALSE ("program_stop")) -> ()
  n350 = Unbundle(w22) -> ("Reference & Errors"=w18:T3, "Reference & Errors"=w17:T3, "Reference & Errors"=w16:T3)
  n351 = Unbundle(w23) -> ("Initialised?"=w21:bool, "Initialised?"=w20:bool, "Initialised?"=w19:bool)
  n352 = Unbundle(w4) -> ("RecordingInProgress"=w1:bool, "refnum out"=w3:refnum<file>, "error out"=w2:errorcluster)  [unwired: 1 out]
  n353 = case shown="True" w1 {
    tunnel: w3 -> [_ w908]
    tunnel: w2 -> [_ w907]
    frame False {
    }
    frame True {
      n354 = Close File(refnum=w908, error in=w907) -> (error out=w909:errorcluster)  [unwired: 1 out]
      n355 = call <vilib>:"Simple Error Handler.vi"("error in (no error)"=w909) -> ()  [unwired: 4 in, 5 out]
    }
  }
  n356 = case shown="True" w21 {
    tunnel: w18 -> [_ w910]
    frame False {
    }
    frame True {
      n357 = Unbundle(w910) -> ("VISA resource name out"=w912:refnum<visa-resource-name>, "error out"=w911:errorcluster)
      n358 = call <instrlib>:"Close.vi"("error in (no error)"=w911, "VISA resource name"=w912) -> ("error out"=w913:errorcluster)  [unwired: 9 in]
      n359 = call <vilib>:"Simple Error Handler.vi"("error in (no error)"=w913) -> ()  [unwired: 4 in, 5 out]
    }
  }
  n360 = case shown="True" w20 {
    tunnel: w17 -> [_ w914]
    frame False {
    }
    frame True {
      n361 = Unbundle(w914) -> ("VISA resource name out"=w916:refnum<visa-resource-name>, "error out"=w915:errorcluster)
      n362 = call <instrlib>:"Close.vi"("error in (no error)"=w915, "VISA resource name"=w916) -> ("error out"=w917:errorcluster)  [unwired: 9 in]
      n363 = call <vilib>:"Simple Error Handler.vi"("error in (no error)"=w917) -> ()  [unwired: 4 in, 5 out]
    }
  }
  n364 = case shown="True" w19 {
    tunnel: w16 -> [_ w918]
    frame False {
    }
    frame True {
      n365 = Unbundle(w918) -> ("VISA resource name out"=w920:refnum<visa-resource-name>, "error out"=w919:errorcluster)
      n366 = call <instrlib>:"Close.vi"("error in (no error)"=w919, "VISA resource name"=w920) -> ("error out"=w921:errorcluster)  [unwired: 9 in]
      n367 = call <vilib>:"Simple Error Handler.vi"("error in (no error)"=w921) -> ()  [unwired: 4 in, 5 out]
    }
  }
